vi "Set Control File Attribute (Version).vi"(8 "error in (no error)":errorcluster, 10 "version":string, 11 "control file refnum in":refnum<file>) -> (0 "error out":errorcluster, 3 "control file refnum out":refnum<file>)   [LabVIEW 2014, in "NIPM_API.lvlib"]
doc: "Modifies the Version package attribute in an unpacked package's control file.\n\nINPUT(s)\n<B>Control file refnum in</B>: This is a file refnum from an unpacked package's control file. Use the Open/Create/Replace File function to open a control file and pass its file refnum to this VI.\n\n<B>Version</B>: This VI writes this version to the Version package attribute in the control file.\n\nOUTPUT(s)\n<B>Control file refnum out</B>: Passes the control file refnum out of this VI."
uses:
  NIPM_API.lvlib
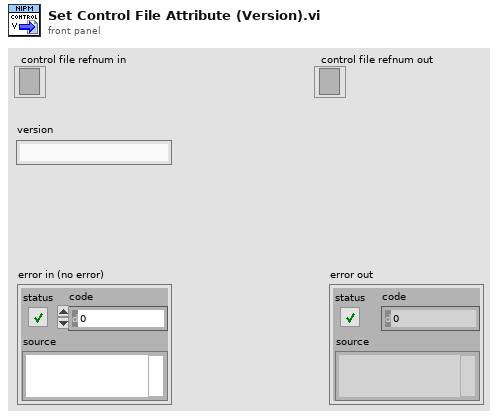
[diagram p1: front panel]
types:
  T1 = enum16{"open", "replace", "create", "open or create", "replace or create", "replace or create with confirmation"}
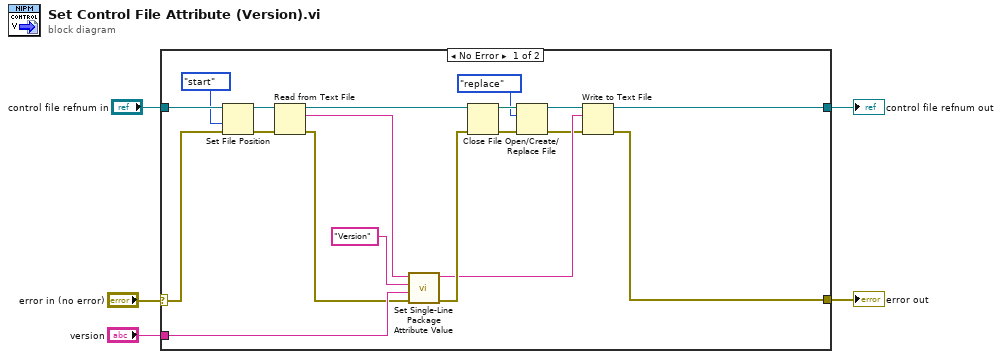
[diagram p0: block diagram]
diagram:
  n1 = case shown="No Error" "error in (no error)" {
    selector: "error in (no error)" -> [w17 w26]
    tunnel: "control file refnum in" -> [w14 w25]
    tunnel: [w18 w25] -> w4
    tunnel: [w19 w26] -> w2
    tunnel: "version" -> [w22 _]
    frame No Error {
      n2 = Set File Position(refnum=w14, from (0:start)=enum16{"start", "end", "current"}."start", error in=w17) -> (refnum out=w13:refnum<file>, error out=w15:errorcluster)  [unwired: 1 in]
      n3 = Read from Text File(file (use dialog)=w13, error in=w15) -> (refnum out=w8:refnum<file>, text=w24:string, error out=w16:errorcluster)  [unwired: 2 in, 1 out]
      n4 = call "Set Single-Line Package Attribute Value.vi"("error in (no error)"=w16, "package attribute value"=w22, "package attribute name"="Version", "package attributes string in"=w24) -> ("error out"=w21:errorcluster, "package attributes string out"=w20:string)  [unwired: 4 in, 2 out]
      n5 = Close File(refnum=w8, error in=w21) -> (path=w7:path, error out=w9:errorcluster)
      n6 = Open/Create/Replace File(file path (use dialog)=w7, error in=w9, operation (0:open)=T1."replace") -> (refnum out=w10:refnum<file>, error out=w11:errorcluster)  [unwired: 3 in, 1 out]
      n7 = Write to Text File(file (use dialog)=w10, text=w20, error in=w11) -> (refnum out=w18:refnum<file>, error out=w19:errorcluster)  [unwired: 1 in, 1 out]
    }
    frame Error {
    }
  }
  "control file refnum out" <- w4
  "error out" <- w2
